vi "Get Error Handling Message Queue.vi"(8 "Error In":errorcluster, 11 "Central Message Handler In":refnum<class "Central Message Handler.lvclass">) -> (0 "Error Out":errorcluster, 2 "Error Handling Message Queue":refnum<queue>, 3 "Central Message Handler Out":refnum<class "Central Message Handler.lvclass">)   [LabVIEW 2019, in "Central Message Handler.lvclass"]
uses:
  Central Message Handler.lvclass
  Process/Public/Controls/Process Message.ctl
  Accessors/Processes Queues Map/Get Processes Queues Map.vi
  Process/Process.lvclass
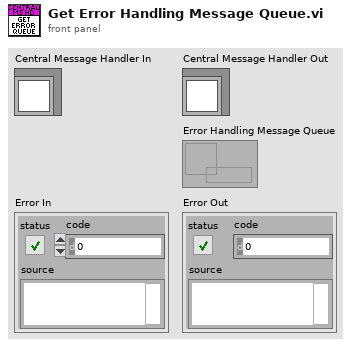
[diagram p1: front panel]
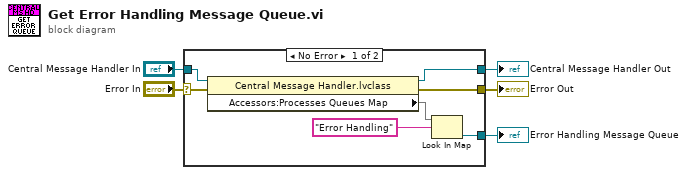
[diagram p0: block diagram]
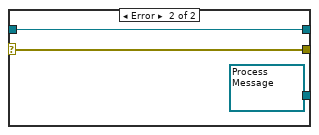
[diagram p2: hidden frame]
diagram:
  n1 = case shown="No Error" "Error In" {
    selector: "Error In" -> [w9 w14]
    tunnel: [w12 w15] -> w5
    tunnel: [w11 w14] -> w4
    tunnel: "Central Message Handler In" -> [w8 w15]
    tunnel: [w6 refnum<queue> refnum ("Accessors:Message Queue")] -> w1
    frame No Error {
      n2 = property class="Central Message Handler.lvclass"(reference=w8, error in=w9) -> (reference out=w12:refnum<class "Central Message Handler.lvclass">, error out=w11:errorcluster, "Accessors:Processes Queues Map"=w10:map{string, refnum<queue>})
      n3 = Look In Map(map=w10, key="Error Handling") -> (value=w6:refnum<queue>)  [unwired: 1 in, 1 out]
    }
    frame Error {
    }
  }
  "Central Message Handler Out" <- w5
  "Error Out" <- w4
  "Error Handling Message Queue" <- w1
